vi "Tool selector (SubVI).vi"(4 "Tips or no tips":bool, 5 "Z, Hight":dbl format="%#_13g", 6 "Obejct length":dbl, 7 "Tool size values":dbl[](array[numeric]), 8 "Assignment -Task - Tool":string) -> (0 "Tool 2":string, 1 "Obejct length out":dbl, 2 "Tool":dbl, 3 "Assignment - Task":string)   [LabVIEW 2024]
doc: "Selecting tool from object length.\nCorrecting height from user input."
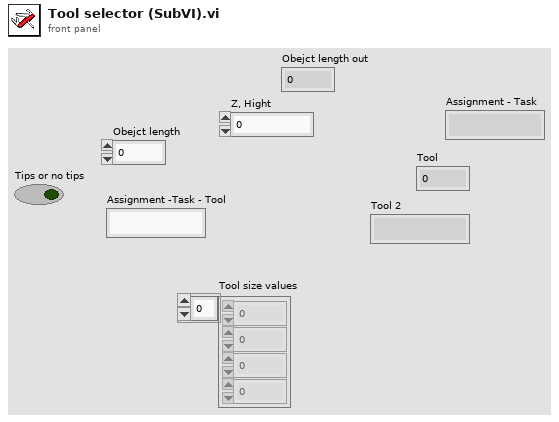
[diagram p1: front panel]
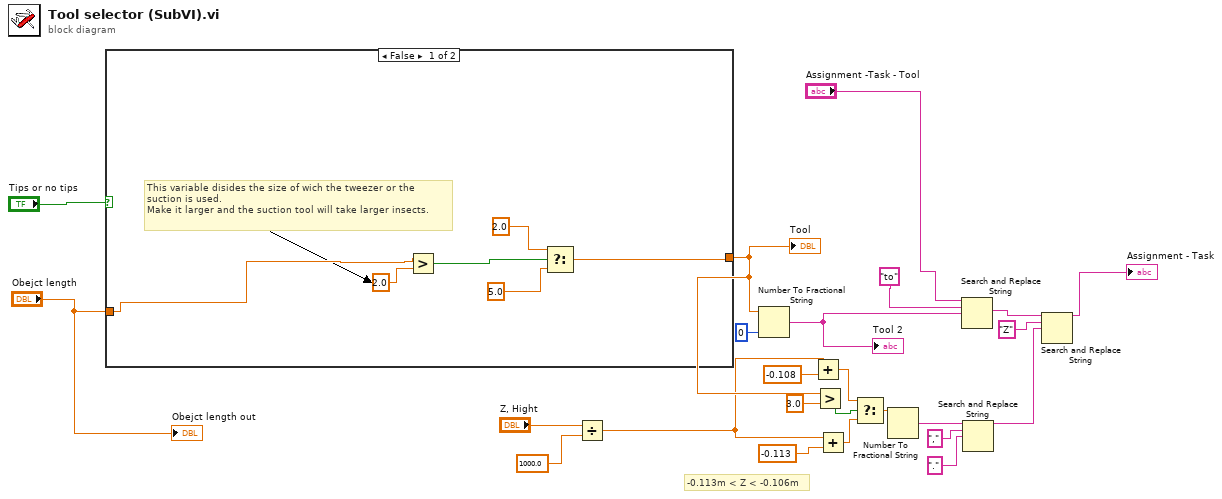
[diagram p0: block diagram]
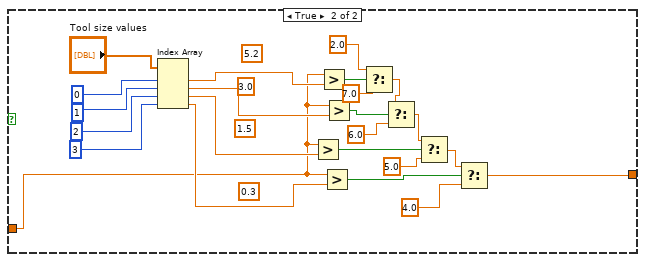
[diagram p2: hidden frame]
diagram:
  # "-0.113m < Z < -0.106m"
  n1 = case shown="False" "Tips or no tips" {
    tunnel: [w26 w43] -> w12
    tunnel: "Obejct length" -> [w25 w31]
    frame False {
      # "This variable disides the size of wich the tweezer or the suction is used.\nMake it larger and the suction tool will take larger insects."
      n2 = Greater?(x=w25, y=2.0) -> (0:w30:bool)
      n3 = Select(t=2.0, s=w30, f=5.0) -> (s? t:f=w26:dbl)
    }
    frame True {
      (unwired) 5.2 ("y")
      (unwired) 3.0 ("y")
      (unwired) 1.5 ("y")
      (unwired) 0.3 ("upper limit")
      n4 = Index Array(array="Tool size values", index #1=0 ("index"), index #2=1 ("index"), index #3=2 ("index"), index #4=3 ("index")) -> (element #1=w32:dbl, element #2=w33:dbl, element #3=w34:dbl, element #4=w35:dbl)
      n5 = Greater?(x=w31, y=w34) -> (0:w46:bool)
      n6 = Greater?(x=w31, y=w32) -> (0:w44:bool)
      n7 = Greater?(x=w31, y=w35) -> (0:w45:bool)
      n8 = Greater?(x=w31, y=w33) -> (0:w48:bool)
      n9 = Select(t=2.0, s=w44, f=7.0) -> (s? t:f=w52:dbl)
      n10 = Select(t=w52, s=w48, f=6.0) -> (s? t:f=w49:dbl)
      n11 = Select(t=w49, s=w46, f=5.0) -> (s? t:f=w47:dbl)
      n12 = Select(t=w47, s=w45, f=4.0) -> (s? t:f=w43:dbl)
    }
  }
  "Tool" <- w12
  n13 = Divide(x="Z, Hight", y=1000.0) -> (x/y=w10:dbl)
  n14 = Number To Fractional String(number=w12, precision (6)=i16 0) -> (F-format string=w24:string)  [unwired: 2 in]
  "Tool 2" <- w24
  n15 = Add(x=w10, y=-0.108) -> (x+y=w7:dbl)
  n16 = Greater?(x=w12, y=3.0) -> (0:w5:bool)
  n17 = Add(x=w10, y=-0.113 ("Z, Hight")) -> (x+y=w6:dbl)
  n18 = Select(t=w7, s=w5, f=w6) -> (s? t:f=w8:dbl)
  n19 = Number To Fractional String(number=w8) -> (F-format string=w15:string)  [unwired: 3 in]
  n20 = Search and Replace String(input string="Assignment -Task - Tool", search string="to", replace string=w24) -> (result string=w14:string)  [unwired: 5 in, 3 out]
  n21 = Search and Replace String(input string=w15, search string=",", replace string="." ("replace string (\"\")")) -> (result string=w4:string)  [unwired: 5 in, 3 out]
  n22 = Search and Replace String(input string=w14, search string="Z", replace string=w4) -> (result string=→"Assignment - Task":string)  [unwired: 5 in, 3 out]
  "Obejct length out" <- "Obejct length"
